vi "OptimalAngle.vi"(10 "Y (feet)":dbl=8.0, 11 "X (feet)":dbl) -> (3 "Angle (degrees)":dbl)   [LabVIEW 2015]
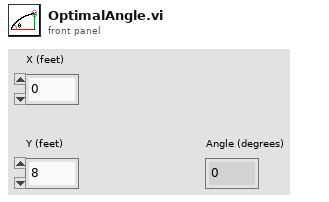
[diagram p1: front panel]
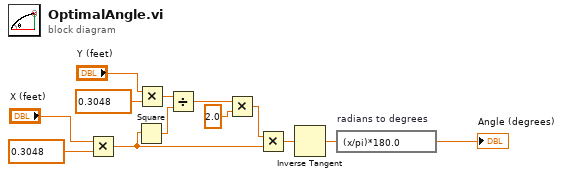
[diagram p0: block diagram]
diagram:
  n1 = Multiply(x="X (feet)", y=0.3048 ("Ft to m")) -> (x*y=w5:dbl)
  n2 = Square(x=w5) -> (x^2=w6:dbl)
  n3 = Multiply(x="Y (feet)", y=0.3048 ("Ft to m")) -> (x*y=w10:dbl)
  n4 = Divide(x=w10, y=w6) -> (x/y=w8:dbl)
  n5 = Multiply(x=w8, y=2.0) -> (x*y=w7:dbl)
  n6 = Multiply(x=w7, y=w5) -> (x*y=w4:dbl)
  n7 = Inverse Tangent(1:w4) -> (0:w3:dbl)
  n8 = expression code="(x/pi)*180.0" "radians to degrees"(w3) -> (→"Angle (degrees)":dbl)
